vi "INVENTORY2sql.vi"() -> ()   [LabVIEW 2015]
uses:
  Controls/STORE_INPUT_NO_CLUSTER.ctl
  Controls/STORE_INPUT_INFORMATION_Cluster.ctl
  <vilib>/addons/database/Connection.llb/DB Tools Open Connec (String).vi
  <vilib>/addons/database/Connection.llb/Conn Execute.vi
  <vilib>/addons/database/Recordset.llb/Rec Destroy - Connection.vi
  <vilib>/addons/database/_DB Variant To Data/Database Variant To Data.xnode
  <vilib>/addons/database/NI_Database_API.lvlib
panel:
  out "error out 5":errorcluster
  out "Numeric":i32
  out "error out 4":errorcluster
  out "error out 3":errorcluster
  out "error out 2":errorcluster
  out "error out":errorcluster
  out "Find Array":i32[](array[numeric])
  out "Input No.":string
  out "Table 2":string[][](table)
  out "ECODE":string
  in  "Input Date":timestamp format="%<%d/%m/%Y>T"
  in  "Browse":path=path "\\\\192.168.1.45\\Du Lieu Kho/Data/Inventory" caption="Path"
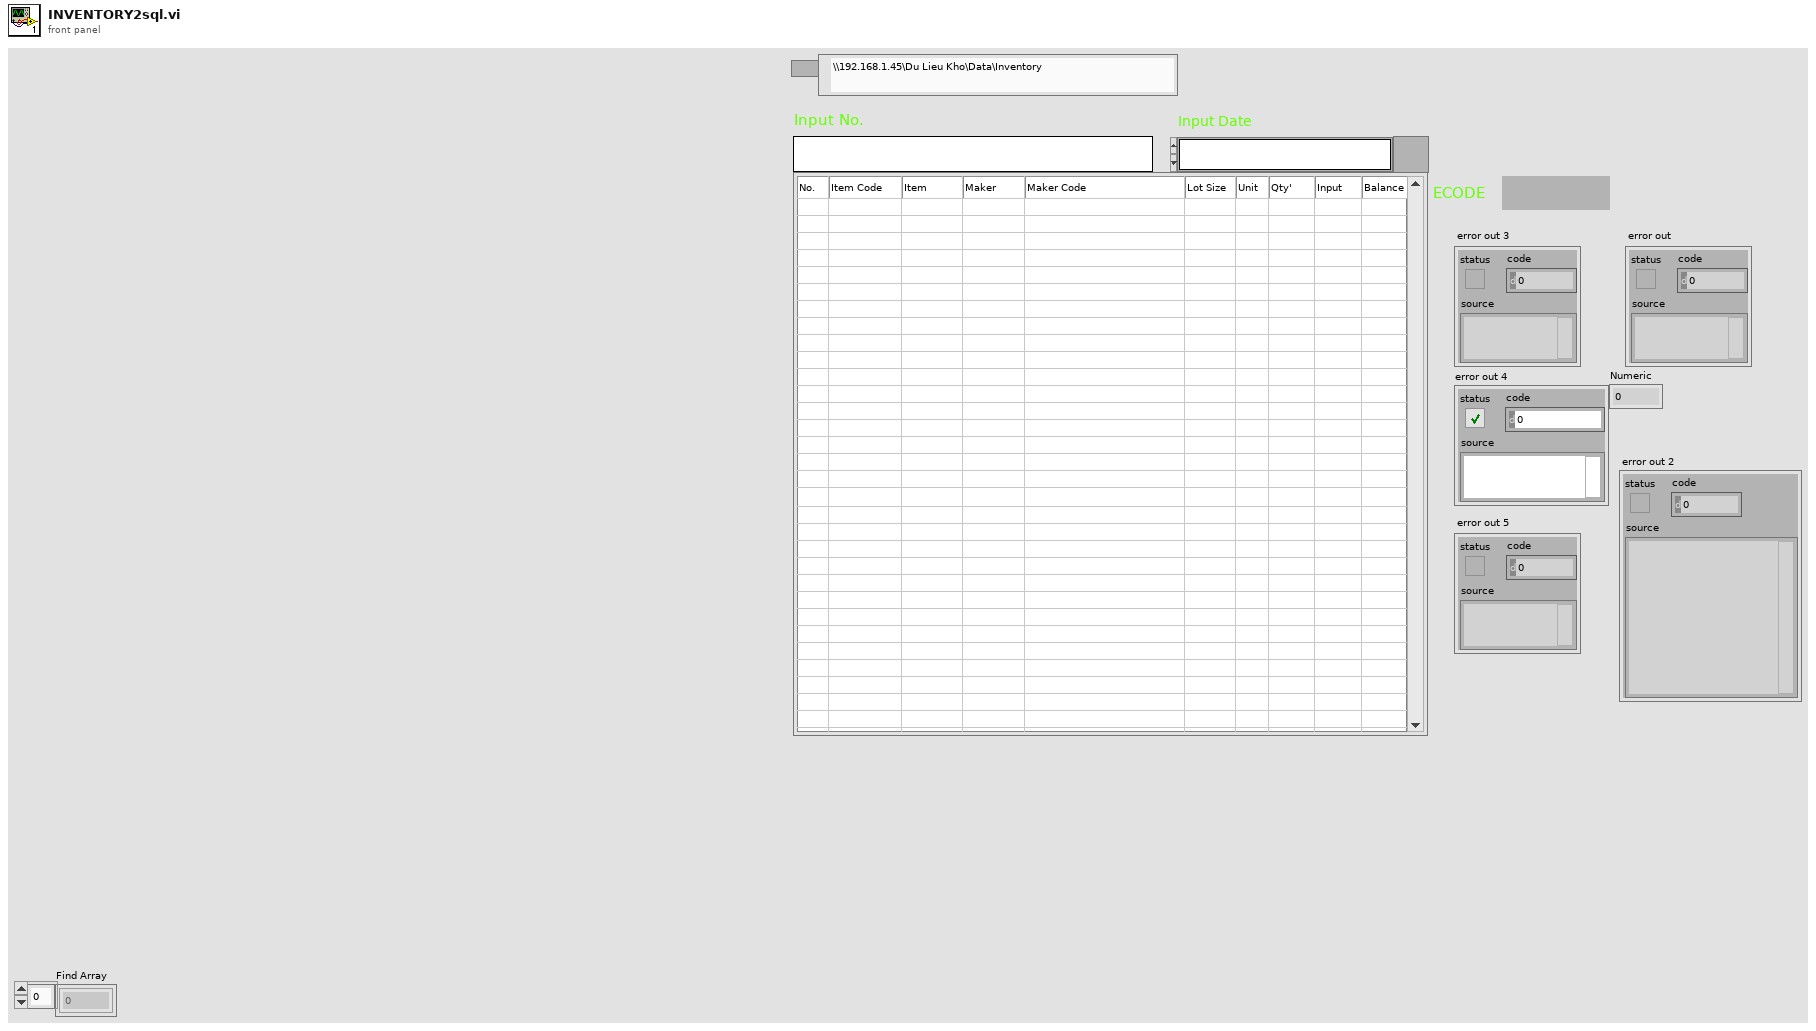
[diagram p1: front panel]
types:
  T1 = typedef "STORE_INPUT_NO_CLUSTER.ctl" = cluster{"NO":dbl, "ITEM_CODE":string, "ITEM":string, "MAKER":string, "MAKER_CODE":string, "LOT_SIZE":dbl, "UNIT":string, "QUANTITY":dbl, "INPUT":dbl, "BALANCE":dbl, "DESTINATION":string, "INVOICE_NO":string}
  T2 = enum16{"open", "replace", "create", "open or create", "replace or create", "replace or create with confirmation"}
  T3 = typedef "STORE_INPUT_INFORMATION_Cluster.ctl" = cluster{"INPUT_NO":string, "INPUT_DATE":timestamp, "ECODE":string}
  T4 = typedef "NI_Database_API.lvlib/Conn ObjectReference.ctl" = refnum<k1>
  T5 = typedef "NI_Database_API.lvlib/Rec ObjectReference.ctl" = refnum<k1>
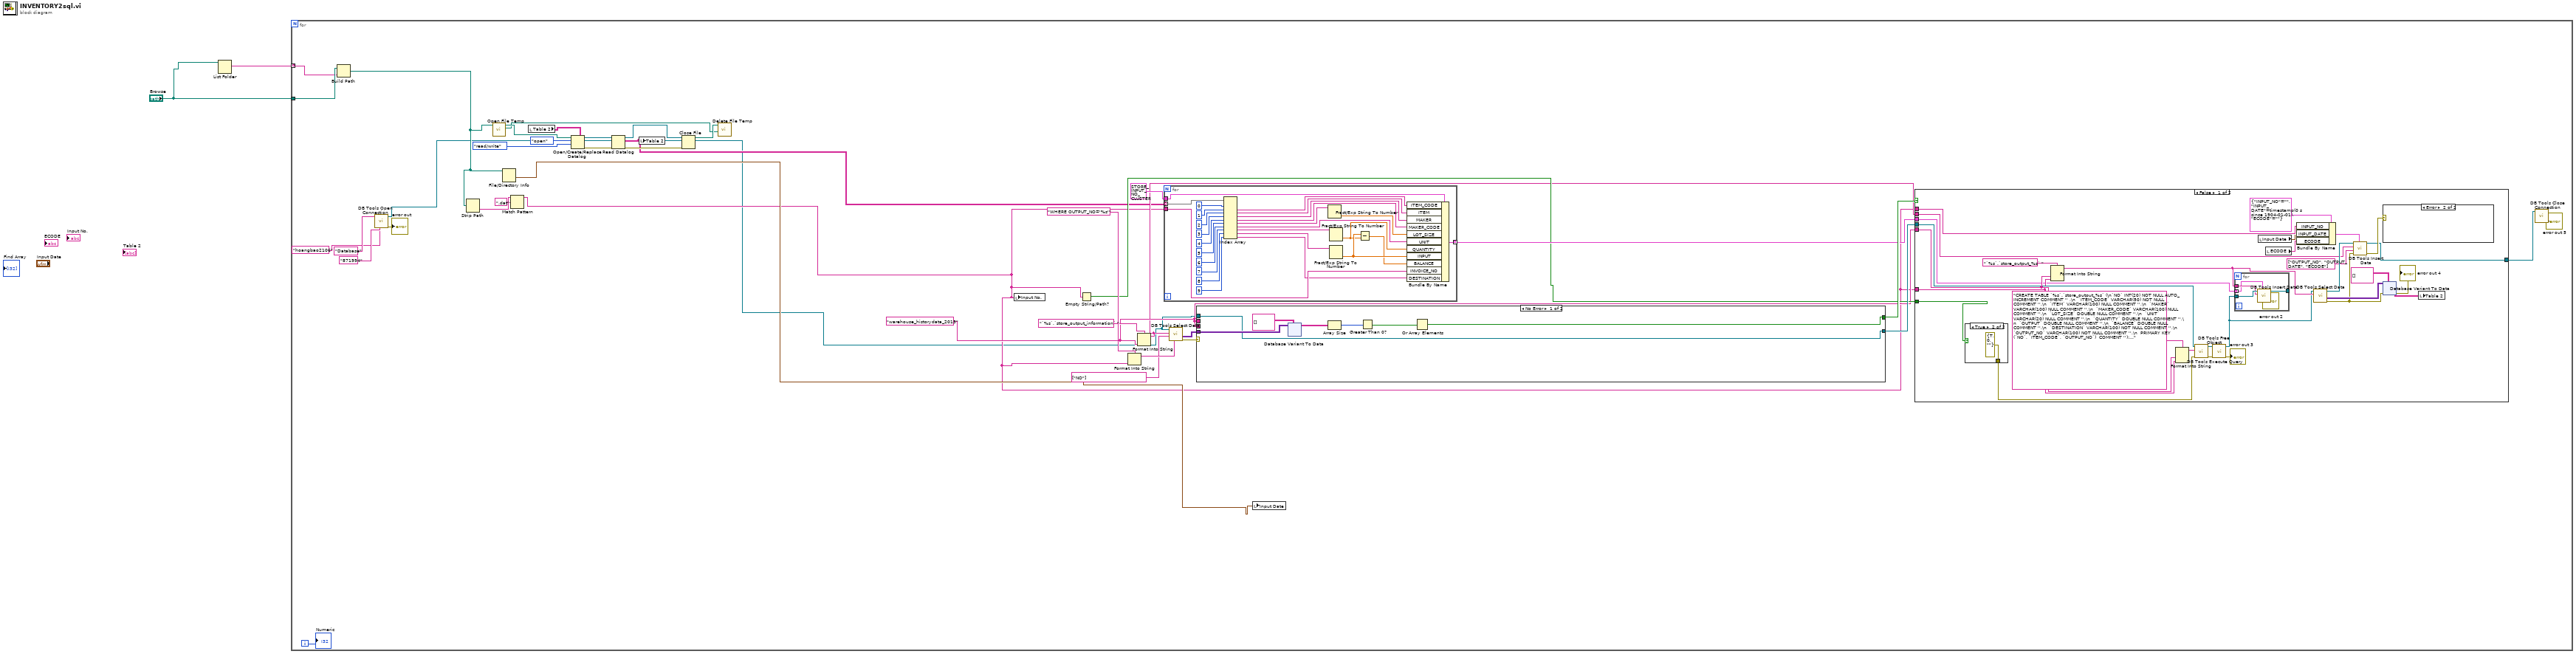
[diagram p0: block diagram]
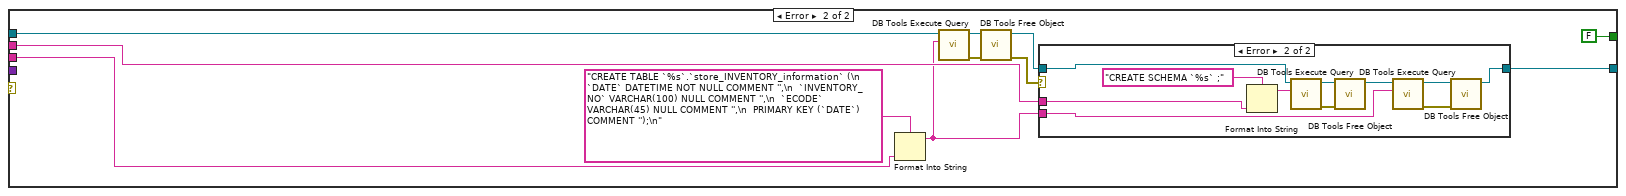
[diagram p2: hidden frame]
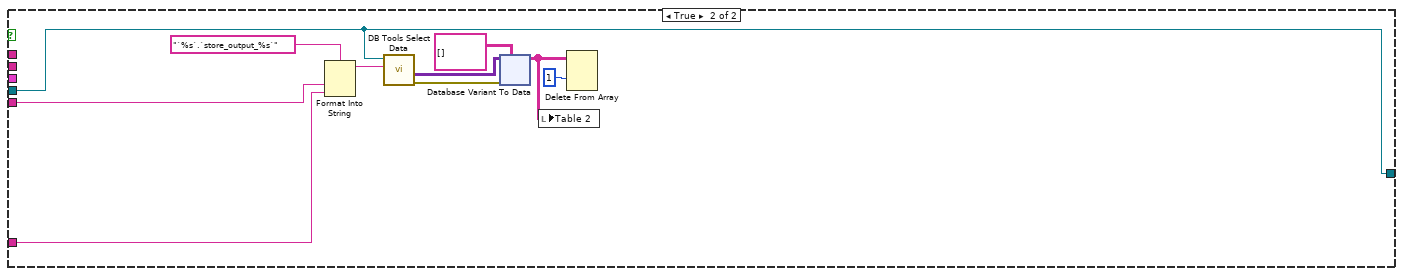
[diagram p6: hidden frame]
diagram:
  n1 = List Folder(path="Browse") -> (filenames=w2:string[])  [unwired: 3 in, 3 out]
  n2 = for {
    tunnel: "Browse" -> [w13]
    tunnel: w2 -> [w12] mode=indexing
    i -> [w10]
    w20 = "warehouse_historydata_2015"
    n3 = Build Path(base path=w13, name or relative path=w12) -> (appended path=w11:path)
    n4 = call-poly <vilib>:"DB Tools Open Connection.vi"("password"="871994" ("userID"), "userID"="hoangbao2106", "connection information"="Database" ("userID")) -> ("error out"=→"error out":errorcluster, "connection reference"=w5:T4)  [unwired: 5 in]
    n5 = Strip Path(path=w11) -> (name=w17:string)  [unwired: 1 out]
    n6 = call "Open File Temp.vi"("Path file"=w11) -> ("Source Path"=w32:path, "Temp path"=w34:path)  [unwired: 7 in, 2 out]
    n7 = File/Directory Info(path=w11) -> (last mod=w18:timestamp)  [unwired: 1 in, 6 out]
    n8 = Match Pattern(string=w17, regular expression=".dat") -> (before substring=w14:string)  [unwired: 1 in, 3 out]
    n9 = local read "Table 2"() -> (w41:string[][])
    n10 = Open/Create/Replace Datalog(5:w41, 9:enum16{"read/write", "read-only", "write-only"}."read/write" ("access (0:read/write)"), 10:T2."open" ("operation (0:open)"), 11:w34) -> (0:w36:errorcluster, 3:w38:refnum<k1>)  [unwired: 2 in, 1 out]
    n11 = Read Datalog(4:w36, 7:w38) -> (0:w35:errorcluster, 2:w15:string[][], 3:w37:refnum<k1>)  [unwired: 1 in]
    n12 = local write "Table 2"(w15) -> ()
    n13 = Close File(refnum=w37, error in=w35) -> (path=w33:path)  [unwired: 1 out]
    n14 = call "Delete File Temp.vi"("Source Path"=w32, "Temp path"=w33) -> ()  [unwired: 8 in, 2 out]
    n15 = local write "Input No."(w14) -> ()
    n16 = Empty String/Path?(string/path=w14) -> (empty?=w22:bool)
    n17 = Format Into String(format string="WHERE OUTPUT_NO='%s'", w14) -> (resulting string=w30:string)  [unwired: 2 in, 1 out]
    n18 = Format Into String(format string="`%s`.`store_output_information` ", w20) -> (resulting string=w19:string)  [unwired: 2 in, 1 out]
    n19 = for {
      tunnel: w15 -> [w67] mode=indexing
      tunnel: T1 {"NO"=0.0, "ITEM_CODE"="", "ITEM"="", "MAKER"="", "MAKER_CODE"="", "LOT_SIZE"=0.0, "UNIT"="", "QUANTITY"=0.0, "INPUT"=0.0, "BALANCE"=0.0, "DESTINATION"="", "INVOICE_NO"=""} -> [w68]
      tunnel: [w47] -> w23 mode=indexing
      tunnel: w14 -> [w46]
      n20 = Index Array(array=w67, index #1=0 ("index"), index #2=1 ("index"), index #3=2 ("index"), index #4=3 ("index"), index #5=4 ("index"), index #6=5 ("index"), index #7=6 ("index"), index #8=7 ("index"), index #9=8 ("index"), index #10=9 ("index")) -> (element #2=w56:string, element #3=w55:string, element #4=w54:string, element #5=w53:string, element #6=w52:string, element #7=w50:string, element #8=w49:string, element #9=w48:string, element #10=w42:string)  [unwired: 1 out]
      n21 = Fract/Exp String To Number(string=w52) -> (number=w51:dbl)  [unwired: 3 in, 1 out]
      n22 = Fract/Exp String To Number(string=w49) -> (number=w44:dbl)  [unwired: 3 in, 1 out]
      n23 = Fract/Exp String To Number(string=w48) -> (number=w45:dbl)  [unwired: 3 in, 1 out]
      n24 = Subtract(x=w45, y=w44) -> (x-y=w43:dbl)
      n25 = Bundle By Name(cluster=w68, "ITEM_CODE"=w56, "ITEM"=w55, "MAKER"=w54, "MAKER_CODE"=w53, "LOT_SIZE"=w51, "UNIT"=w50, "QUANTITY"=w44, "INPUT"=w45, "BALANCE"=w43, "INVOICE_NO"=w46, "DESTINATION"=w42) -> (w47:T1)
    }
    n26 = call <vilib>:"DB Tools Select Data.vi"("condition"=w30, "columns"=string[] ["NO"], "table"=w19, "connection reference"=w5) -> ("error out"=w26:errorcluster, "data"=w29:variant[][])  [unwired: 2 in, 1 out]
    n27 = case shown="No Error" w26 {
      tunnel: w29 -> [w75 _]
      tunnel: [w70 FALSE] -> w27
      tunnel: w5 -> [w69 w127]
      tunnel: [w69 w123] -> w25
      tunnel: w20 -> [_ w125]
      tunnel: w20 -> [_ w121]
      frame No Error {
        n28 = xnode "Database Variant To Data"("database variant"=w75, "type"=string[][] []) -> ("data"=w73:string[][])  [unwired: 1 in, 1 out]
        n29 = Array Size(array=w73) -> (size(s)=w72:i32[])
        n30 = Greater Than 0?(x=w72) -> (x > 0?=w71:bool[])
        n31 = Or Array Elements(Boolean array=w71) -> (logical OR=w70:bool)
      }
      frame Error {
        n32 = Format Into String(format string="CREATE TABLE `%s`.`store_INVENTORY_information` (\n  `DATE` DATETIME NOT NULL COMMENT '',\n  `INVENTORY_NO` VARCHAR(100) NULL COMMENT '',\n  `ECODE` VARCHAR(45) NULL COMMENT '',\n  PRIMARY KEY (`DATE`)  COMMENT '');\n", w121) -> (resulting string=w120:string)  [unwired: 2 in, 1 out]
        n33 = call-poly <vilib>:"DB Tools Execute Query.vi"("SQL query"=w120, "connection reference"=w127) -> ("error out"=w129:errorcluster, "recordset reference"=w130:T5)  [unwired: 6 in]
        n34 = call-poly <vilib>:"DB Tools Free Object.vi"("error in (no error)"=w129, "recordset reference"=w130) -> ("error out"=w126:errorcluster, "connection reference"=w124:T4)  [unwired: 8 in]
        n35 = case shown="Error" w126 {
          tunnel: w124 -> [w131 w142]
          tunnel: w125 -> [_ w140]
          tunnel: w120 -> [_ w134]
          tunnel: [w131 w133] -> w123
          frame No Error {
          }
          frame Error {
            n36 = Format Into String(format string="CREATE SCHEMA `%s` ;" ("SQL query"), w140) -> (resulting string=w132:string)  [unwired: 2 in, 1 out]
            n37 = call-poly <vilib>:"DB Tools Execute Query.vi"("SQL query"=w132, "connection reference"=w142) -> ("error out"=w138:errorcluster, "recordset reference"=w139:T5)  [unwired: 6 in]
            n38 = call-poly <vilib>:"DB Tools Free Object.vi"("error in (no error)"=w138, "recordset reference"=w139) -> ("connection reference"=w135:T4)  [unwired: 8 in, 1 out]
            n39 = call-poly <vilib>:"DB Tools Execute Query.vi"("SQL query"=w134, "connection reference"=w135) -> ("error out"=w137:errorcluster, "recordset reference"=w136:T5)  [unwired: 6 in]
            n40 = call-poly <vilib>:"DB Tools Free Object.vi"("error in (no error)"=w137, "recordset reference"=w136) -> ("connection reference"=w133:T4)  [unwired: 8 in, 1 out]
          }
        }
      }
    }
    n41 = local write "Input Date"(w18) -> ()
    n42 = case shown="False" w27 {
      tunnel: w25 -> [w171 w231]
      tunnel: w20 -> [w166 w225]
      tunnel: w14 -> [w165 w226]
      tunnel: [w154 w231] -> w4
      tunnel: w23 -> [w164 _]
      tunnel: w19 -> [w157 _]
      tunnel: w14 -> [w153 _]
      tunnel: w22 -> [w147 _]
      frame False {
        n43 = case shown="True" w147 {
          tunnel: [_ errorcluster {"status"=TRUE, "code"=0, "source"=""} ("error constant")] -> w146
          frame False {
          }
          frame True {
          }
        }
        n44 = Format Into String(format string="`%s`.`store_output_%s` " ("SQL query"), w166, w165) -> (resulting string=w160:string)  [unwired: 2 in, 1 out]
        n45 = Format Into String(format string="CREATE TABLE `%s`.`store_output_%s` (\n`NO` INT(20) NOT NULL AUTO_INCREMENT COMMENT '' ,\n  `ITEM_CODE` VARCHAR(50) NOT NULL COMMENT '',\n  `ITEM` VARCHAR(100) NULL COMMENT '',\n  `MAKER` VARCHAR(100) NULL COMMENT '',\n  `MAKER_CODE` VARCHAR(100) NULL COMMENT '',\n  `LOT_SIZE` DOUBLE NULL COMMENT '',\n  `UNIT` VARCHAR(20) NULL COMMENT '',\n  `QUANTITY` DOUBLE NULL COMMENT '',\n  `OUTPUT` DOUBLE NULL COMMENT '',\n  `BALANCE` DOUBLE NULL COMMENT '',\n  `DESTINATION` VARCHAR(100) NOT NULL COMMENT '',\n  `OUTPUT_NO` VARCHAR(100) NOT NULL COMMENT '',\n  PRIMARY KEY (`NO`, `ITEM_CODE`, `OUTPUT_NO`)  COMMENT '');\n" ("SQL query"), w166, w165) -> (resulting string=w159:string)  [unwired: 2 in, 1 out]
        n46 = call-poly <vilib>:"DB Tools Execute Query.vi"("error in (no error)"=w146, "SQL query"=w159, "connection reference"=w171) -> ("error out"=w168:errorcluster, "recordset reference"=w169:T5)  [unwired: 5 in]
        n47 = call-poly <vilib>:"DB Tools Free Object.vi"("error in (no error)"=w168, "recordset reference"=w169) -> ("error out"=→"error out 3":errorcluster, "connection reference"=w145:T4)  [unwired: 8 in]
        n48 = for {
          tunnel: w145 -> [w221]
          tunnel: w160 -> [w220]
          tunnel: w164 -> [w219] mode=indexing
          tunnel: [w218] -> _
          n49 = call <vilib>:"DB Tools Insert Data.vi"("data"=w219, "table"=w220, "connection reference"=w221) -> ("error out"=→"error out 2":errorcluster, "connection reference out"=w218:T4)  [unwired: 7 in]
        }
        n50 = local read "Input Date"() -> (w152:timestamp)
        n51 = local read "ECODE"() -> (w151:string)
        n52 = Bundle By Name(cluster=T3 {"INPUT_NO"="", "INPUT_DATE"=timestamp(0 s since 1904-01-01), "ECODE"=""} ("INVOICE_INFORMATION_Cluster"), "INPUT_NO"=w153, "INPUT_DATE"=w152, "ECODE"=w151) -> (w150:T3)
        n53 = call <vilib>:"DB Tools Select Data.vi"("table"=w160, "connection reference"=w145) -> ("error out"=w156:errorcluster, "data"=w163:variant[][], "connection reference out"=w158:T4)  [unwired: 4 in]
        n54 = call <vilib>:"DB Tools Insert Data.vi"("data"=w150, "error in (no error)"=w156, "columns"=string[] ["OUTPUT_NO", "OUTPUT_DATE", "ECODE"], "table"=w157, "connection reference"=w158) -> ("error out"=w155:errorcluster, "connection reference out"=w154:T4)  [unwired: 5 in]
        n55 = case shown="Error" w155 {
          frame No Error {
          }
          frame Error {
          }
        }
        n56 = xnode "Database Variant To Data"("database variant"=w163, "error in (no error)"=w156, "type"=string[][] []) -> ("data"=w161:string[][], "error out"=→"error out 4":errorcluster)
        n57 = local write "Table 2"(w161) -> ()
      }
      frame True {
        n58 = Format Into String(format string="`%s`.`store_output_%s`", w225, w226) -> (resulting string=w224:string)  [unwired: 2 in, 1 out]
        n59 = call <vilib>:"DB Tools Select Data.vi"("table"=w224, "connection reference"=w231) -> ("error out"=w228:errorcluster, "data"=w230:variant[][])  [unwired: 4 in, 1 out]
        n60 = xnode "Database Variant To Data"("database variant"=w230, "error in (no error)"=w228, "type"=string[][] []) -> ("data"=w223:string[][])  [unwired: 1 out]
        n61 = local write "Table 2"(w223) -> ()
        n62 = Delete From Array(array=w223, index (row)=1) -> ()  [unwired: 2 in, 2 out]
      }
    }
    n63 = call <vilib>:"DB Tools Close Connection.vi"("connection reference"=w4) -> ("error out"=→"error out 5":errorcluster)  [unwired: 6 in]
    "Numeric" <- w10
  }
